vi "Filter.vi"(1 "Array":cdb[](array[numeric]) format="%.2f") -> (0 "Filtered Array":cdb[](array[numeric]) format="%.2f")   [LabVIEW 2009]
uses:
  <vilib>/Analysis/2dsp.llb/Inverse Complex FFT.vi
  <vilib>/Analysis/2dsp.llb/Complex FFT.vi
  <vilib>/Analysis/NI_AALPro.lvlib
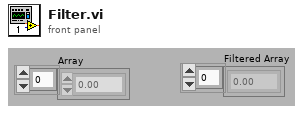
[diagram p1: front panel]
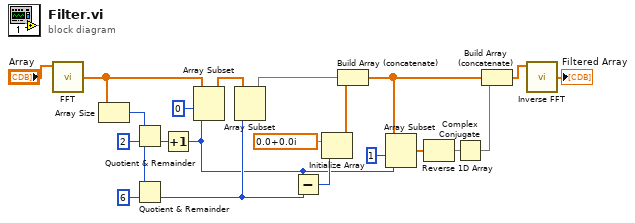
[diagram p0: block diagram]
diagram:
  n1 = call-poly <vilib>:"FFT.vi"("X"="Array") -> ("FFT {X}"=w3:cdb[])  [unwired: 9 in, 1 out]
  n2 = Array Size(array=w3) -> (size(s)=w15:i32)
  n3 = Quotient & Remainder(x=w15, y=2) -> (floor(x/y)=w2:i32)  [unwired: 1 out]
  n4 = Quotient & Remainder(x=w15, y=6) -> (floor(x/y)=w17:i32)  [unwired: 1 out]
  n5 = Increment(x=w2) -> (x+1=w7:i32)
  n6 = Array Subset(array=w3, index=0 ("indice"), length=w7) -> (w4:cdb[])
  n7 = Array Subset(array=w4, length=w17) -> (w9:cdb[])  [unwired: 1 in]
  n8 = Subtract(x=w7, y=w17) -> (x-y=w20:i32)
  n9 = Initialize Array(cdb 0.0+0.0i ("Element Data"), w20) -> (w10:cdb[])
  n10 = Build Array (concatenate)(w9, w10) -> (w11:cdb[])
  n11 = Array Subset(array=w11, index=1 ("Array Index"), length=w7) -> (w12:cdb[])
  n12 = Reverse 1D Array(array=w12) -> (reversed array=w13:cdb[])
  n13 = Complex Conjugate(1:w13) -> (0:w21:cdb[])
  n14 = Build Array (concatenate)(w11, w21) -> (w14:cdb[])
  n15 = call-poly <vilib>:"Inverse FFT.vi"("FFT {X}"=w14) -> ("X"=→"Filtered Array":cdb[])  [unwired: 9 in, 1 out]
